vi "Infinite Message Manager.vi"(0 "Father of all uServices in":refnum<class "Father of all uServices.lvclass">, 5 "Consumer Case Selector":variant, 7 "Data":variant, 9 "Tau parameter":string, 11 "error in (no error)":errorcluster, 12 "Infinite Message Selector":T1=enum."Check") -> (4 "Father of all uServices out":refnum<class "Father of all uServices.lvclass">, 6 "Exists?":bool, 15 "error out":errorcluster)   [LabVIEW 2026, in "TALOS.lvlib" / "Father of all uServices.lvlib" / "Father of all uServices.lvclass"]
doc: "This VI is useful to manage (start, check, stop and flush) some Consumer Cases, to be enqueued periodically. The period is specified in Tau Parameter, which must be the name of a parameter present in the configuration ini file (if not specified, 1 s is assumed as default). Note that at the closure of a uService, all the infinite messages present will be flushed."
uses:
  Father of all uServices.lvclass
  Ancestor/Ancestor/Infinite Message Selector.ctl
  Father of all uServices Messages/Consumer Msg/Consumer Msg.lvclass
  C:/LabVIEW Code/TALOS/builds/Actor Framework PPL/Actor Framework.lvlibp/1abvi3w/vi.lib/ActorFramework/Message/Message.lvclass
  <userlib>/_OpenG.lib/lvdata/lvdata.llb/openg_variant.lvlib
  Ancestor/Ancestor/Ancestor.lvclass
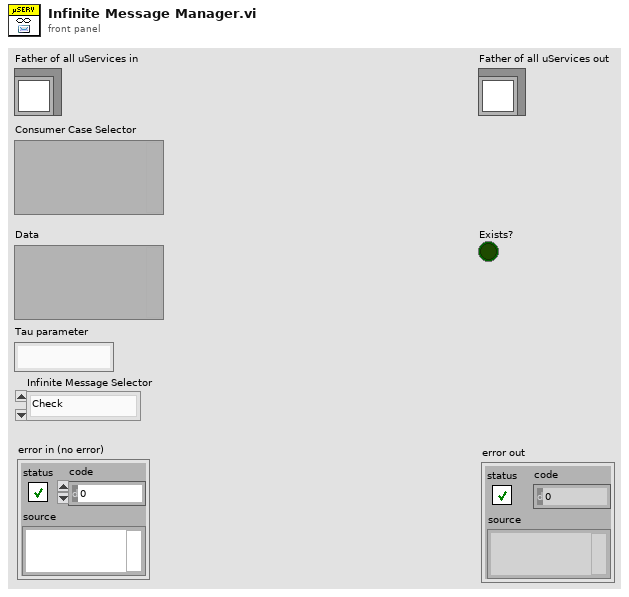
[diagram p1: front panel]
types:
  T1 = typedef "TALOS.lvlib/Ancestor.lvlib/Ancestor.lvclass/Infinite Message Selector.ctl" = enum16{"Start", "Stop", "Check", "Flush (Stop all)", "Init"}
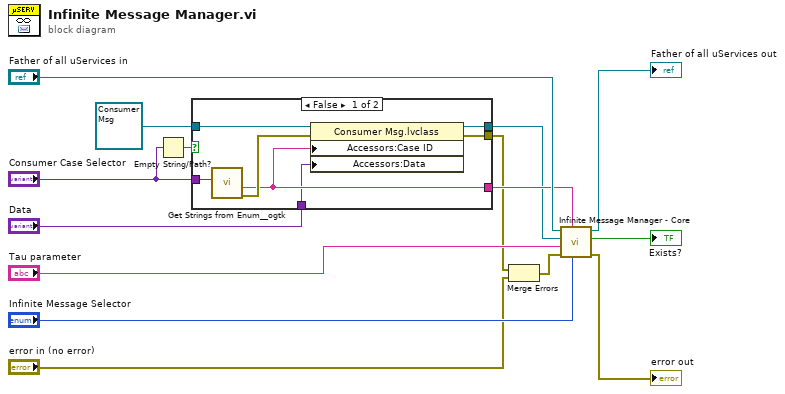
[diagram p0: block diagram]
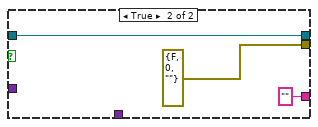
[diagram p2: hidden frame]
diagram:
  n1 = Empty String/Path?(string/path="Consumer Case Selector") -> (empty?=w3:bool)
  n2 = case shown="False" w3 {
    tunnel: "Consumer Case Selector" -> [w22 _]
    tunnel: [w20 "" ("String Value")] -> w9
    tunnel: "Data" -> [w19 _]
    tunnel: [w18 w25] -> w7
    tunnel: [w17 errorcluster {"status"=FALSE, "code"=0, "source"=""} ("error out")] -> w6
    tunnel: refnum<class "Consumer Msg.lvclass"> refnum ("TALOS.lvlib:Father of all uServices.lvlib:Consumer Msg.lvclass") -> [w16 w25]
    frame False {
      n3 = call <userlib>:"Get Strings from Enum__ogtk.vi"("Enum"=w22) -> ("error out"=w21:errorcluster, "String Value"=w20:string)  [unwired: 7 in, 2 out]
      n4 = property class="Consumer Msg.lvclass"(reference=w16, error in=w21, "Accessors:Case ID"=w20, "Accessors:Data"=w19) -> (reference out=w18:refnum<class "Consumer Msg.lvclass">, error out=w17:errorcluster)
    }
    frame True {
    }
  }
  n5 = Merge Errors(w6, "error in (no error)") -> (w4:errorcluster)
  n6 = call-dynamic "Infinite Message Manager - Core.vi"("Infinite Message Selector"="Infinite Message Selector", "Msg ID"=w9, "error in (no error)"=w4, "Tau parameter"="Tau parameter", "Actor Framework:Message"=w7, "Ancestor in"="Father of all uServices in") -> ("error out"=→"error out":errorcluster, "Exists?"=→"Exists?":bool, "Ancestor out"=→"Father of all uServices out":refnum<class "Father of all uServices.lvclass">)  [unwired: 3 in]
